vi "WhyWouldAnyOneNeedToMakeANewVIToStoreAndUseABool.vi"(11 "Boolean":bool) -> (3 "Boolean 2":bool)   [LabVIEW 2015]
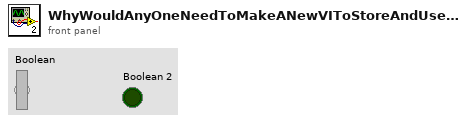
[diagram p1: front panel]
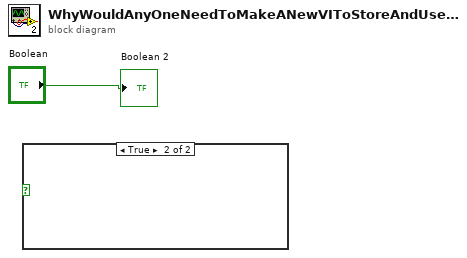
[diagram p0: block diagram]
diagram:
  n1 = case shown="True" {
    selector: _ -> [_ _]
    frame False {
    }
    frame True {
    }
  }
  "Boolean 2" <- "Boolean"
